vi "Measurement Convertor.vi"(2 "Measurement":string, 3 "Expression":string) -> (0 "Temp":dbl, 1 "Value":u32)   [LabVIEW 2023]
uses:
  <vilib>/regexp/Match Regular Expression.xnode
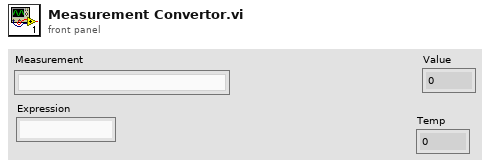
[diagram p1: front panel]
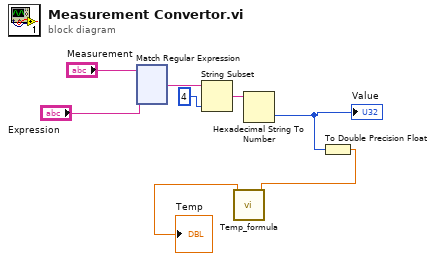
[diagram p0: block diagram]
diagram:
  n1 = xnode "Match Regular Expression"("input string"="Measurement", "regular expression"="Expression") -> ("after match"=w7:string)  [unwired: 4 in, 4 out]
  n2 = String Subset(string=w7, length (rest)=4 ("length (rest)")) -> (substring=w5:string)  [unwired: 1 in]
  n3 = Hexadecimal String To Number(string=w5) -> (number=w3:u32)  [unwired: 2 in, 1 out]
  "Value" <- w3
  n4 = To Double Precision Float(number=w3) -> (double precision float=w2:dbl)
  n5 = call "Temp_formula.vi"("NTCin"=w2) -> ("TempOut"=→"Temp":dbl)  [unwired: 10 in]
